vi "WPI_CANJaguar_ScheduleDefaultStatus.vi"(8 "error in (no error)":errorcluster, 11 "CAN Jaguar Ref Out in":T1={"DeviceStatus"={"status"=FALSE, "code"=0, "source"=""}, "Type"=enum."PWM", "PWM"={"PWM Channel"=enum."PWM 0", "DeadBand"={"Name"="", "maxPositivePwm"=0, "minPositivePwm"=0, "centerPwm"=0, "maxNegativePwm"=0, "minNegativePwm"=0, "angularRange"=0}}, "CAN"={"Device Number"=0, "SetOutput VI Ref"=variant(enum8{"Percent VBus", "Current", "Speed", "Position", "Voltage"} enum."Percent VBus"), "GetOutput VI Ref"=variant(refnum<k1> refnum), "Enable VI Ref"=variant(dbl 0.0), "Disable VI Ref"=variant(enum8{"Percent VBus", "Speed", "Position", "Slave", "Unchanged / Invalid", "Voltage Compensation", "Current", "Motion Profile"} enum."Percent VBus"), "Data"=variant}, "Invert"=FALSE}) -> (0 "error out":errorcluster, 3 "CAN Jaguar Ref Out out":T1={"DeviceStatus"={"status"=FALSE, "code"=0, "source"=""}, "Type"=enum."PWM", "PWM"={"PWM Channel"=enum."PWM 0", "DeadBand"={"Name"="", "maxPositivePwm"=0, "minPositivePwm"=0, "centerPwm"=0, "maxNegativePwm"=0, "minNegativePwm"=0, "angularRange"=0}}, "CAN"={"Device Number"=0, "SetOutput VI Ref"=variant(enum8{"Percent VBus", "Current", "Speed", "Position", "Voltage"} enum."Percent VBus"), "GetOutput VI Ref"=variant(refnum<k1> refnum), "Enable VI Ref"=variant(dbl 0.0), "Disable VI Ref"=variant(enum8{"Percent VBus", "Speed", "Position", "Slave", "Unchanged / Invalid", "Voltage Compensation", "Current", "Motion Profile"} enum."Percent VBus"), "Data"=variant}, "Invert"=FALSE})   [LabVIEW 2016]
uses:
  <vilib>/Rock Robotics/WPI/MotorControl/WPI_MotorControlDeviceRef.ctl
  <vilib>/Rock Robotics/WPI/MotorControl/WPI_MotorControlType.ctl
  <vilib>/Rock Robotics/SystemInterfaces/DIO/FPGA_DIOPWMChannel.ctl
  <vilib>/Rock Robotics/WPI/PWM/WPI_PWMDeadband.ctl
  <vilib>/Rock Robotics/WPI/ThirdParty/CanMotor/CAN Jaguar/SubVIs/WPI_CANJaguar_StatusChannelSelect.ctl
  <vilib>/Rock Robotics/WPI/ThirdParty/CanMotor/CAN Jaguar/SubVIs/WPI_CANJaguar_StatusSelect.ctl
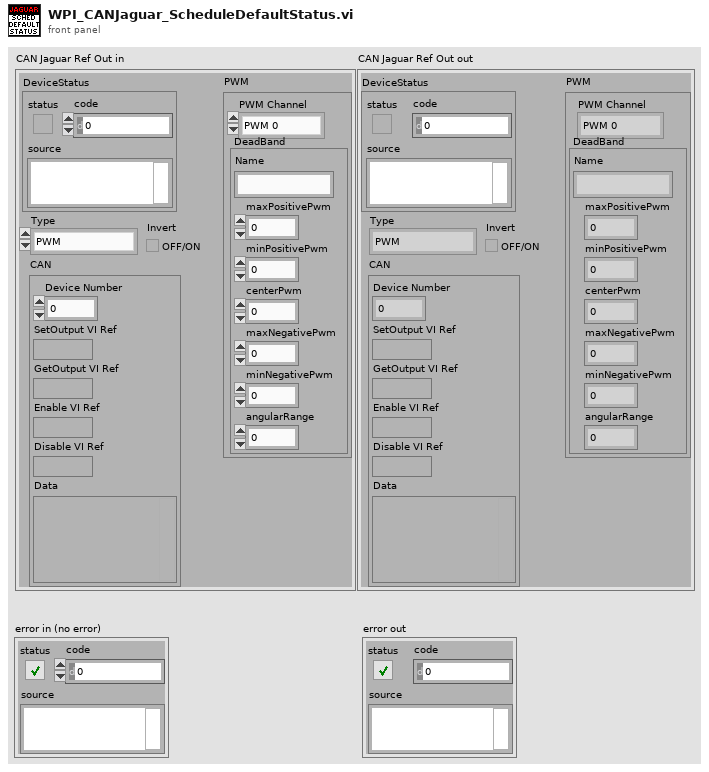
[diagram p1: front panel]
types:
  T1 = typedef "WPI_MotorControlDeviceRef.ctl" = cluster{"DeviceStatus":errorcluster, "Type":T2, "PWM":cluster{"PWM Channel":T3, "DeadBand":T4}, "CAN":cluster{"Device Number":u8, "SetOutput VI Ref":variant, "GetOutput VI Ref":variant, "Enable VI Ref":variant, "Disable VI Ref":variant, "Data":variant}, "Invert":bool}
  T2 = typedef "WPI_MotorControlType.ctl" = enum16{"PWM", "CAN"}
  T3 = typedef "FPGA_DIOPWMChannel.ctl" = enum8{"PWM 0", "PWM 1", "PWM 2", "PWM 3", "PWM 4", "PWM 5", "PWM 6", "PWM 7", "PWM 8", "PWM 9", "PWM MXP 0", "PWM MXP 1", "PWM MXP 2", "PWM MXP 3", "PWM MXP 4", "PWM MXP 5", "PWM MXP 6", "PWM MXP 7", "PWM MXP 8", "PWM MXP 9", "Invalid"}
  T4 = typedef "WPI_PWMDeadband.ctl" = cluster{"Name":string, "maxPositivePwm":i32, "minPositivePwm":i32, "centerPwm":i32, "maxNegativePwm":i32, "minNegativePwm":i32, "angularRange":u16}
  T5 = typedef "WPI_CANJaguar_StatusSelect.ctl" = enum16{"Output Percent VBus", "Output Voltage", "Bus Voltage", "Current", "Temperature", "Position", "Speed", "Limit Switches", "Faults", "Fault Counters", "Power Cycle"}
  T6 = typedef "WPI_CANJaguar_StatusChannelSelect.ctl" = enum16{"Periodic Status Channel 1", "Periodic Status Channel 2", "Periodic Status Channel 3", "Periodic Status Channel 4", "On Demand Status"}
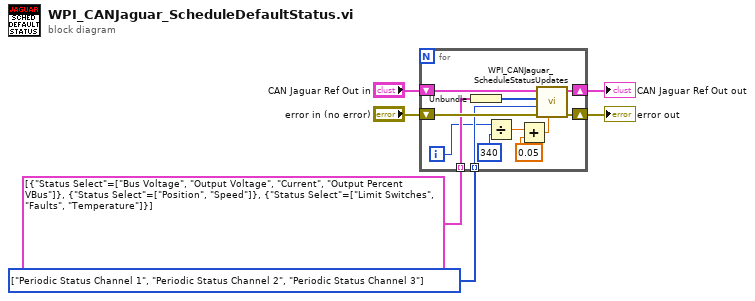
[diagram p0: block diagram]
diagram:
  w2 = T6[] [enum."Periodic Status Channel 1", enum."Periodic Status Channel 2", enum."Periodic Status Channel 3"] items=["Periodic Status Channel 1", "Periodic Status Channel 2", "Periodic Status Channel 3", "Periodic Status Channel 4", "On Demand Status"]
  n1 = for {
    shift-right: [w16] -> w5
    shift-left: "CAN Jaguar Ref Out in" -> [w18]
    shift-right: [w15] -> w6
    shift-left: "error in (no error)" -> [w17]
    tunnel: w2 -> [w14] mode=indexing
    tunnel: cluster{"Status Select":T5[]}[] [{"Status Select"=[enum."Bus Voltage", enum."Output Voltage", enum."Current", enum."Output Percent VBus"]}, {"Status Select"=[enum."Position", enum."Speed"]}, {"Status Select"=[enum."Limit Switches", enum."Faults", enum."Temperature"]}] -> [w13] mode=indexing
    i -> [w11]
    n2 = Unbundle(w13) -> ("Status Select"=w12:T5[])
    n3 = Divide(x=w11, y=340) -> (x/y=w9:dbl)
    n4 = Add(x=w9, y=0.05 ("Update Period (s)")) -> (x+y=w7:dbl)
    n5 = call <vilib>:"WPI_CANJaguar_ScheduleStatusUpdates.vi"("Update Period (s)"=w7, "error in (no error)"=w17, "Status Channel Select"=w14, "Status Select"=w12, "CAN Jaguar Ref"=w18) -> ("error out"=w15:errorcluster, "CAN Jaguar Ref Out"=w16:T1)  [unwired: 5 in]
  }
  "error out" <- w6
  "CAN Jaguar Ref Out out" <- w5
